vi "load.vi"(8 "error in (no error)":errorcluster, 10 "child node in":refnum<k20>, 11 "Analog_Input (in)":refnum<class "Analog_Input.lvclass">) -> (0 "error out":errorcluster, 2 "child node out":refnum<k20>, 3 "Analog_Input":refnum<class "Analog_Input.lvclass">)   [LabVIEW 2014, in "Analog_Input.lvclass"]
uses:
  Analog_Input.lvclass
  Analog_Input.lvclass/Analog_Input.ctl
  Globals.vi
  <vilib>/xml/Close Reference(Node).vi
  <resource>/objmgr/DOMUserDefRef.rc
  <vilib>/xml/NI_XML.lvlib
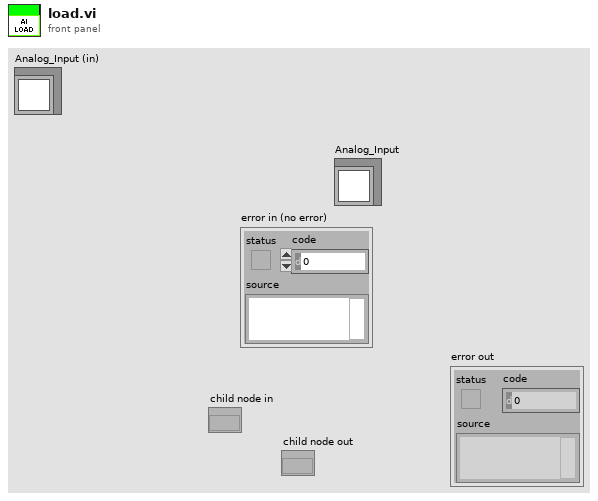
[diagram p1: front panel]
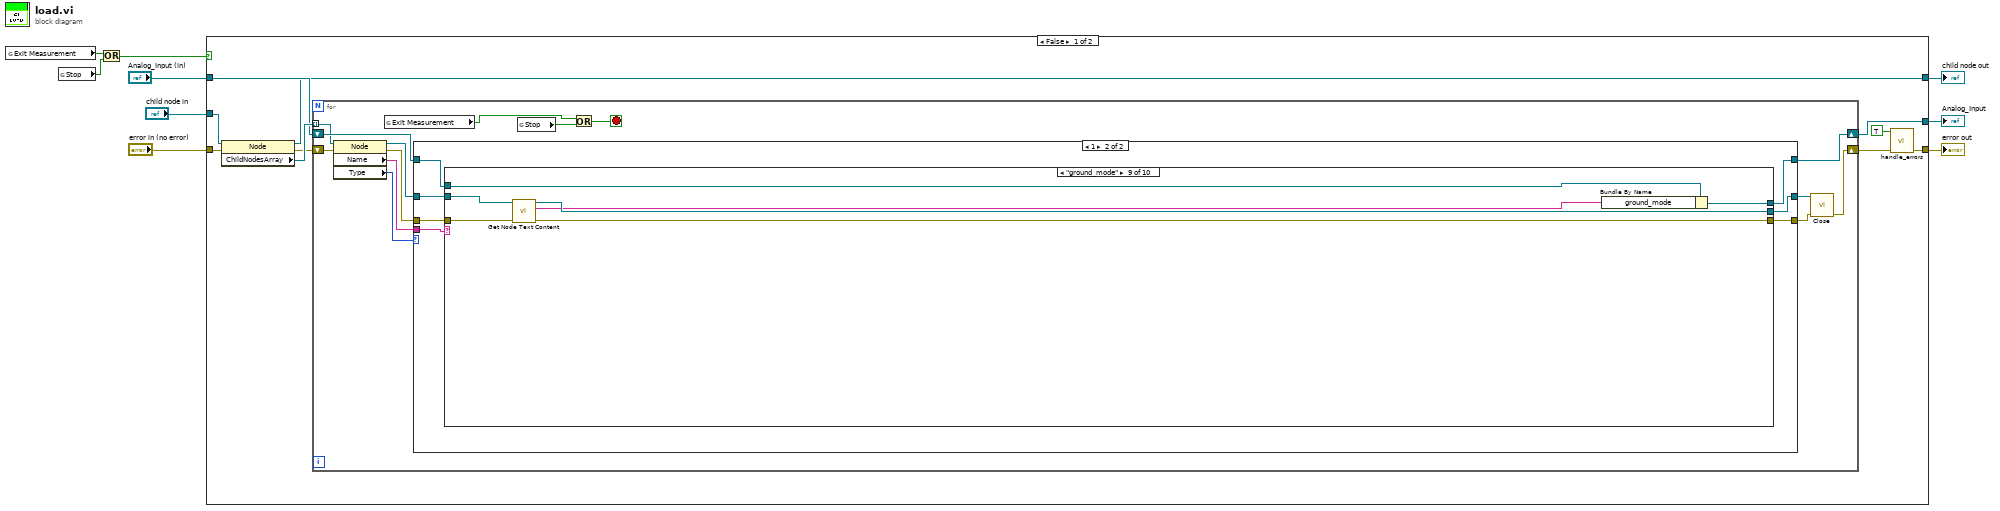
[diagram p0: block diagram]
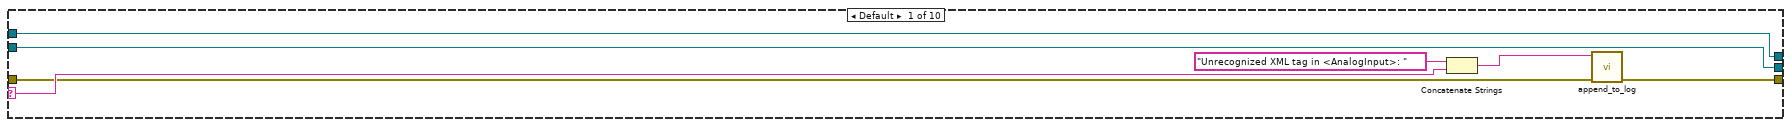
[diagram p3: hidden frame]
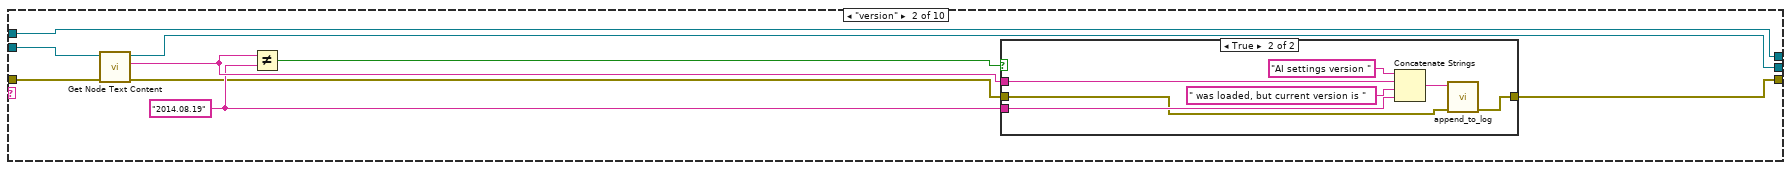
[diagram p4: hidden frame]
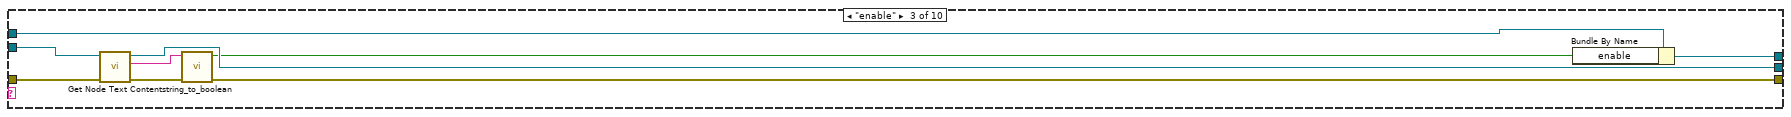
[diagram p6: hidden frame]
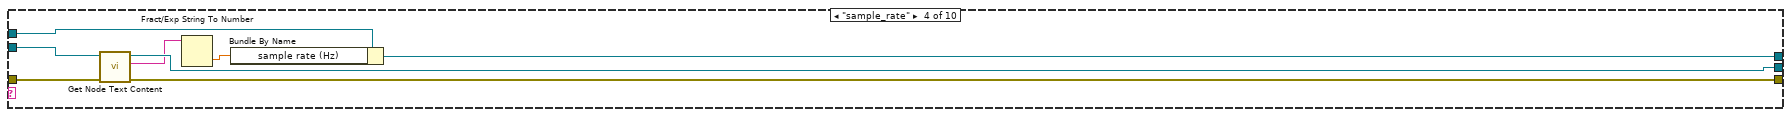
[diagram p7: hidden frame]
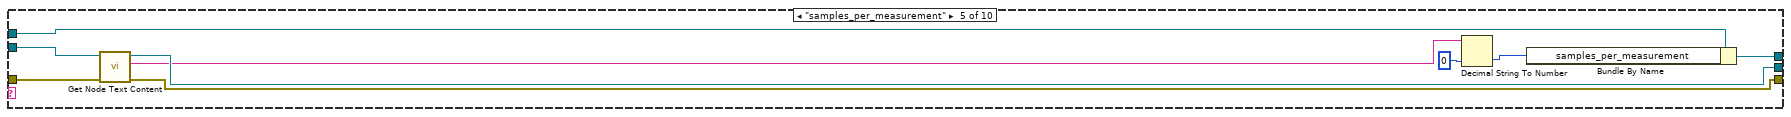
[diagram p8: hidden frame]
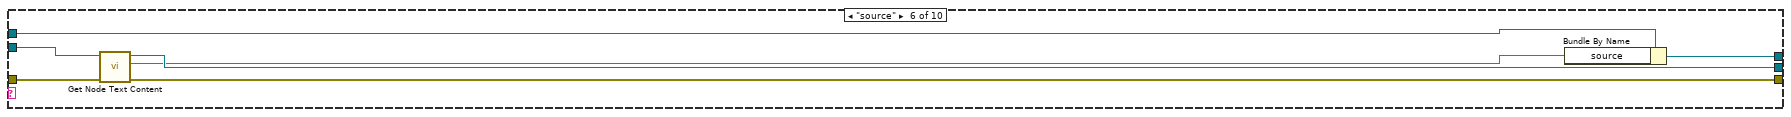
[diagram p9: hidden frame]
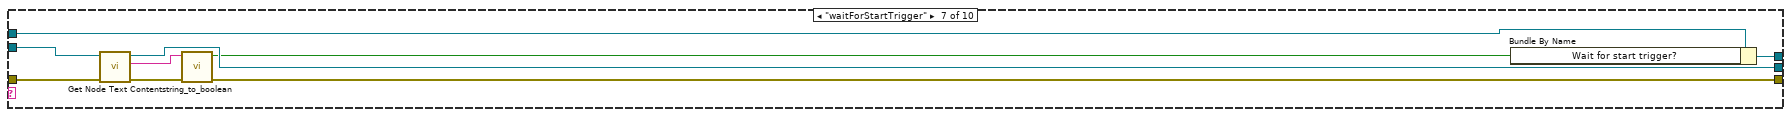
[diagram p10: hidden frame]
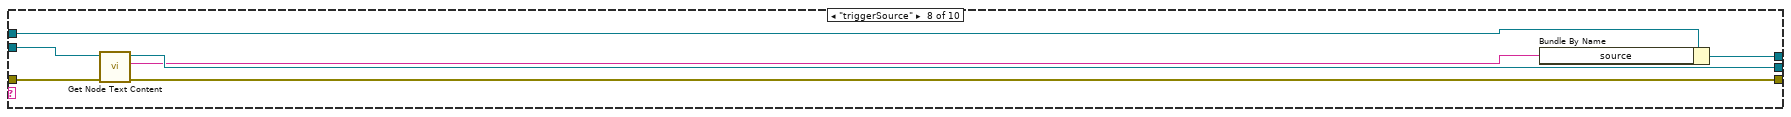
[diagram p11: hidden frame]
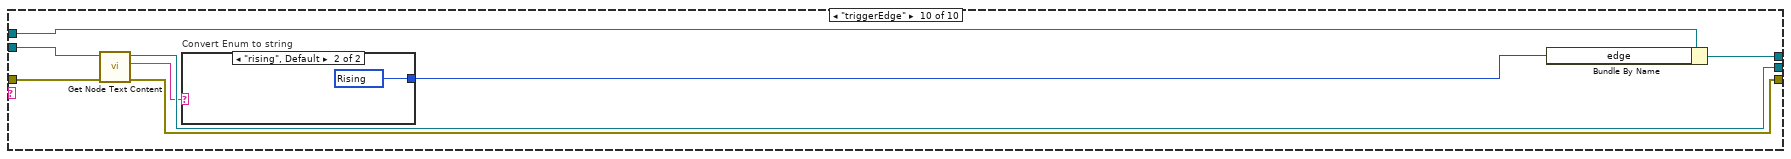
[diagram p12: hidden frame]
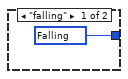
[diagram p13: hidden frame]
diagram:
  n1 = global read "Globals.vi" "Exit Measurement"() -> (w9:bool)
  n2 = global read "Globals.vi" "Stop"() -> (w8:bool)
  n3 = Or(x=w9, y=w8) -> (x .or. y?=w7:bool)
  n4 = case shown="False" w7 {
    tunnel: [w18 w136] -> w5
    tunnel: "error in (no error)" -> [w19 w136]
    tunnel: "Analog_Input (in)" -> [w13 w135]
    tunnel: [w12 w135] -> w1
    tunnel: "child node in" -> [w11 w134]
    tunnel: [w10 w134] -> w3
    frame False {
      n5 = property class="Node"(reference=w11, error in=w19) -> (reference out=w10:refnum<k20>, error out=w16:errorcluster, "ChildNodesArray"=w17:refnum<k20>[])
      n6 = for {
        tunnel: w17 -> [w24] mode=indexing
        shift-right: [w30] -> w12
        shift-left: w13 -> [w31]
        shift-right: [w27] -> w15
        shift-left: w16 -> [w25]
        stop <- w20 stop-if-true
        n7 = property class="Node"(reference=w24, error in=w25) -> (reference out=w32:refnum<k20>, error out=w28:errorcluster, "Name"=w33:string, "Type"=w23:i32)
        n8 = global read "Globals.vi" "Exit Measurement"() -> (w22:bool)
        n9 = case shown="1" w23 {
          tunnel: w33 -> [_ w43]
          tunnel: w32 -> [w36 w42]
          tunnel: w31 -> [w34 w41]
          tunnel: [w34 w40] -> w30
          tunnel: [w36 w39] -> w29
          tunnel: w28 -> [w35 w38]
          tunnel: [w35 w37] -> w26
          frame Default {
          }
          frame 1 {
            n10 = case shown="\"ground_mode\"" w43 {
              selector: w43 -> [w46 _ _ _ _ _ _ _ _ _]
              tunnel: w42 -> [w49 w54 w75 w81 w90 w97 w106 w113 w120 w128]
              tunnel: w41 -> [w50 w53 w73 w84 w93 w100 w109 w116 w123 w131]
              tunnel: [w50 w53 w72 w83 w92 w99 w108 w115 w122 w130] -> w40
              tunnel: [w49 w52 w76 w82 w91 w98 w107 w114 w121 w129] -> w39
              tunnel: w38 -> [w45 w55 w74 w80 w89 w96 w105 w112 w119 w127]
              tunnel: [w44 w51 w68 w79 w88 w95 w102 w111 w118 w126] -> w37
              frame Default {
                n11 = Concatenate Strings("Unrecognized XML tag in <AnalogInput>: " ("string"), w46) -> (w47:string)
                n12 = call "append_to_log.vi"("error in"=w45, "string"=w47) -> ("error out"=w44:errorcluster)  [unwired: 9 in]
              }
              frame "version" {
                w57 = "2014.08.19" ("y")
                n13 = call <vilib>:"Get Node Text Content.vi"("error in (no error)"=w55, "node in"=w54) -> ("error out"=w56:errorcluster, "node text"=w58:string, "node out"=w52:refnum<k20>)  [unwired: 7 in]
                n14 = Not Equal?(x=w58, y=w57) -> (x != y?=w59:bool)
                n15 = case shown="True" w59 {
                  tunnel: w58 -> [_ w66]
                  tunnel: w57 -> [_ w64]
                  tunnel: w56 -> [w60 w62]
                  tunnel: [w60 w61] -> w51
                  frame False {
                  }
                  frame True {
                    n16 = Concatenate Strings("AI settings version " ("string"), w66, " was loaded, but current version is " ("string"), w64) -> (w63:string)
                    n17 = call "append_to_log.vi"("error in"=w62, "string"=w63) -> ("error out"=w61:errorcluster)  [unwired: 9 in]
                  }
                }
              }
              frame "enable" {
                n18 = call <vilib>:"Get Node Text Content.vi"("error in (no error)"=w74, "node in"=w75) -> ("error out"=w70:errorcluster, "node text"=w71:string, "node out"=w76:refnum<k20>)  [unwired: 7 in]
                n19 = call "string_to_boolean.vi"("error in"=w70, "string"=w71) -> ("error out"=w68:errorcluster, "boolean"=w69:bool)  [unwired: 8 in]
                n20 = Bundle By Name(cluster=w73, "enable"=w69) -> (w72:refnum<class "Analog_Input.lvclass">)
              }
              frame "sample_rate" {
                n21 = call <vilib>:"Get Node Text Content.vi"("error in (no error)"=w80, "node in"=w81) -> ("error out"=w79:errorcluster, "node text"=w78:string, "node out"=w82:refnum<k20>)  [unwired: 7 in]
                n22 = Fract/Exp String To Number(string=w78) -> (number=w77:dbl)  [unwired: 3 in, 1 out]
                n23 = Bundle By Name(cluster=w84, "sample rate (Hz)"=w77) -> (w83:refnum<class "Analog_Input.lvclass">)
              }
              frame "samples_per_measurement" {
                n24 = call <vilib>:"Get Node Text Content.vi"("error in (no error)"=w89, "node in"=w90) -> ("error out"=w88:errorcluster, "node text"=w87:string, "node out"=w91:refnum<k20>)  [unwired: 7 in]
                n25 = Decimal String To Number(string=w87, default (0L)=0 ("default (0 I32)")) -> (number=w85:i32)  [unwired: 1 in, 1 out]
                n26 = Bundle By Name(cluster=w93, "samples_per_measurement"=w85) -> (w92:refnum<class "Analog_Input.lvclass">)
              }
              frame "source" {
                n27 = call <vilib>:"Get Node Text Content.vi"("error in (no error)"=w96, "node in"=w97) -> ("error out"=w95:errorcluster, "node text"=w94:string, "node out"=w98:refnum<k20>)  [unwired: 7 in]
                n28 = Bundle By Name(cluster=w100, "source"=w94) -> (w99:refnum<class "Analog_Input.lvclass">)
              }
              frame "waitForStartTrigger" {
                n29 = call <vilib>:"Get Node Text Content.vi"("error in (no error)"=w105, "node in"=w106) -> ("error out"=w103:errorcluster, "node text"=w104:string, "node out"=w107:refnum<k20>)  [unwired: 7 in]
                n30 = call "string_to_boolean.vi"("error in"=w103, "string"=w104) -> ("error out"=w102:errorcluster, "boolean"=w101:bool)  [unwired: 8 in]
                n31 = Bundle By Name(cluster=w109, "Wait for start trigger?"=w101) -> (w108:refnum<class "Analog_Input.lvclass">)
              }
              frame "triggerSource" {
                n32 = call <vilib>:"Get Node Text Content.vi"("error in (no error)"=w112, "node in"=w113) -> ("error out"=w111:errorcluster, "node text"=w110:string, "node out"=w114:refnum<k20>)  [unwired: 7 in]
                n33 = Bundle By Name(cluster=w116, "source"=w110) -> (w115:refnum<class "Analog_Input.lvclass">)
              }
              frame "ground_mode" {
                n34 = call <vilib>:"Get Node Text Content.vi"("error in (no error)"=w119, "node in"=w120) -> ("error out"=w118:errorcluster, "node text"=w117:string, "node out"=w121:refnum<k20>)  [unwired: 7 in]
                n35 = Bundle By Name(cluster=w123, "ground_mode"=w117) -> (w122:refnum<class "Analog_Input.lvclass">)
              }
              frame "triggerEdge" {
                n36 = call <vilib>:"Get Node Text Content.vi"("error in (no error)"=w127, "node in"=w128) -> ("error out"=w126:errorcluster, "node text"=w125:string, "node out"=w129:refnum<k20>)  [unwired: 7 in]
                n37 = case "Convert Enum to string" shown="\"rising\", Default" w125 {
                  tunnel: [w132 w133] -> w124
                  frame "falling" {
                    w132 = 10171 items=["Rising"=10280, "Falling"=10171] ("edge")
                  }
                  frame "rising", Default {
                    w133 = 10280 items=["Rising"=10280, "Falling"=10171] ("edge")
                  }
                }
                n38 = Bundle By Name(cluster=w131, "edge"=w124) -> (w130:refnum<class "Analog_Input.lvclass">)
              }
            }
          }
        }
        n39 = global read "Globals.vi" "Stop"() -> (w21:bool)
        n40 = Or(x=w22, y=w21) -> (x .or. y?=w20:bool)
        n41 = call-poly <vilib>:"Close.vi"("error in (no error)"=w26, "node"=w29) -> ("error out"=w27:errorcluster)  [unwired: 7 in]
      }
      n42 = call "handle_errors.vi"("Exit Operation"=TRUE, "error in (no error)"=w15) -> ("error out"=w18:errorcluster)  [unwired: 13 in]
    }
    frame True {
    }
  }
  "error out" <- w5
  "child node out" <- w3
  "Analog_Input" <- w1
